vi "HatchManipulatorControl.Vi"(0 "Extend":bool, 1 "Slide":bool, 2 "Grip":bool, 3 "Pneumatics":T18={"Shifter"={"DevStatus"={"status"=FALSE, "code"=0, "source"=""}, "Pneumatics Control Module"=0, "Forward Solenoid Channel"=enum."Invalid", "Reverse Solenoid Channel"=enum."Invalid"}, "Compressor"={"DevStatus"={"status"=FALSE, "code"=0, "source"=""}, "Pneumatics Control Module"=0}, "Hatch Grip"={"DevStatus"={"status"=FALSE, "code"=0, "source"=""}, "Pneumatics Control Module"=0, "Forward Solenoid Channel"=enum."Invalid", "Reverse Solenoid Channel"=enum."Invalid"}, "Hatch Extend"={"DevStatus"={"status"=FALSE, "code"=0, "source"=""}, "Pneumatics Control Module"=0, "Forward Solenoid Channel"=enum."Invalid", "Reverse Solenoid Channel"=enum."Invalid"}, "Manipulator Slide"={"DevStatus"={"status"=FALSE, "code"=0, "source"=""}, "Pneumatics Control Module"=0, "Forward Solenoid Channel"=enum."Invalid", "Reverse Solenoid Channel"=enum."Invalid"}, "Hatch Floor Intake"={"DevStatus"={"status"=FALSE, "code"=0, "source"=""}, "Pneumatics Control Module"=0, "Forward Solenoid Channel"=enum."Invalid", "Reverse Solenoid Channel"=enum."Invalid"}}, 4 "RobotConfig":T1={"Motors"={"DriveRightPrimary"={"CAN Address"=1, "Invert"=FALSE, "InvertSensor"=FALSE, "Unit Conversion Factor"=0.0, "Brake Mode"=enum."Override to Brake", "Reverse Limt Switch Mode"=enum."Normally Closed", "Forward Limt Swith Mode"=enum."Normally Closed", "PWM Channel"=enum."Invalid", "Motor Controller Type"=enum."Talon SRX", "Peak Current (A)"=0, "Continuous Current (A)"=0, "Peak Duration (ms)"=0, "Current Limit Enable"=FALSE}, "DriveRightSecondary"={"CAN Address"=2, "Invert"=FALSE, "InvertSensor"=FALSE, "Unit Conversion Factor"=0.0, "Brake Mode"=enum."Override to Brake", "Reverse Limt Switch Mode"=enum."Normally Closed", "Forward Limt Swith Mode"=enum."Normally Closed", "PWM Channel"=enum."Invalid", "Motor Controller Type"=enum."Talon SRX", "Peak Current (A)"=0, "Continuous Current (A)"=0, "Peak Duration (ms)"=0, "Current Limit Enable"=FALSE}, "DriveLeftPrimary"={"CAN Address"=3, "Invert"=FALSE, "InvertSensor"=FALSE, "Unit Conversion Factor"=0.0, "Brake Mode"=enum."Override to Brake", "Reverse Limt Switch Mode"=enum."Normally Closed", "Forward Limt Swith Mode"=enum."Normally Closed", "PWM Channel"=enum."Invalid", "Motor Controller Type"=enum."Talon SRX", "Peak Current (A)"=0, "Continuous Current (A)"=0, "Peak Duration (ms)"=0, "Current Limit Enable"=FALSE}, "DriveLeftSecondary"={"CAN Address"=4, "Invert"=FALSE, "InvertSensor"=FALSE, "Unit Conversion Factor"=0.0, "Brake Mode"=enum."Override to Brake", "Reverse Limt Switch Mode"=enum."Normally Closed", "Forward Limt Swith Mode"=enum."Normally Closed", "PWM Channel"=enum."Invalid", "Motor Controller Type"=enum."Talon SRX", "Peak Current (A)"=0, "Continuous Current (A)"=0, "Peak Duration (ms)"=0, "Current Limit Enable"=FALSE}, "RearClimb"={"CAN Address"=8, "Invert"=FALSE, "InvertSensor"=FALSE, "Unit Conversion Factor"=0.0, "Brake Mode"=enum."Override to Brake", "Reverse Limt Switch Mode"=enum."Normally Closed", "Forward Limt Swith Mode"=enum."Normally Closed", "PWM Channel"=enum."Invalid", "Motor Controller Type"=enum."Talon SRX", "Peak Current (A)"=0, "Continuous Current (A)"=0, "Peak Duration (ms)"=0, "Current Limit Enable"=FALSE}, "Front Climb"={"CAN Address"=7, "Invert"=FALSE, "InvertSensor"=FALSE, "Unit Conversion Factor"=0.0, "Brake Mode"=enum."Override to Brake", "Reverse Limt Switch Mode"=enum."Normally Closed", "Forward Limt Swith Mode"=enum."Normally Closed", "PWM Channel"=enum."Invalid", "Motor Controller Type"=enum."Talon SRX", "Peak Current (A)"=0, "Continuous Current (A)"=0, "Peak Duration (ms)"=0, "Current Limit Enable"=FALSE}, "Climb Drive"={"CAN Address"=5, "Invert"=FALSE, "InvertSensor"=FALSE, "Unit Conversion Factor"=0.0, "Brake Mode"=enum."Override to Brake", "Reverse Limt Switch Mode"=enum."Normally Closed", "Forward Limt Swith Mode"=enum."Normally Closed", "PWM Channel"=enum."Invalid", "Motor Controller Type"=enum."Talon SRX", "Peak Current (A)"=0, "Continuous Current (A)"=0, "Peak Duration (ms)"=0, "Current Limit Enable"=FALSE}, "Shoulder1"={"CAN Address"=6, "Invert"=FALSE, "InvertSensor"=FALSE, "Unit Conversion Factor"=0.0, "Brake Mode"=enum."Override to Brake", "Reverse Limt Switch Mode"=enum."Normally Closed", "Forward Limt Swith Mode"=enum."Normally Closed", "PWM Channel"=enum."Invalid", "Motor Controller Type"=enum."Talon SRX", "Peak Current (A)"=0, "Continuous Current (A)"=0, "Peak Duration (ms)"=0, "Current Limit Enable"=FALSE}, "Shoulder2"={"CAN Address"=9, "Invert"=FALSE, "InvertSensor"=FALSE, "Unit Conversion Factor"=0.0, "Brake Mode"=enum."Override to Brake", "Reverse Limt Switch Mode"=enum."Normally Closed", "Forward Limt Swith Mode"=enum."Normally Closed", "PWM Channel"=enum."Invalid", "Motor Controller Type"=enum."Talon SRX", "Peak Current (A)"=0, "Continuous Current (A)"=0, "Peak Duration (ms)"=0, "Current Limit Enable"=FALSE}, "Wrist"={"CAN Address"=10, "Invert"=FALSE, "InvertSensor"=FALSE, "Unit Conversion Factor"=0.0, "Brake Mode"=enum."Override to Brake", "Reverse Limt Switch Mode"=enum."Disabled", "Forward Limt Swith Mode"=enum."Disabled", "PWM Channel"=enum."Invalid", "Motor Controller Type"=enum."Talon SRX", "Peak Current (A)"=0, "Continuous Current (A)"=0, "Peak Duration (ms)"=0, "Current Limit Enable"=FALSE}, "Extension"={"CAN Address"=11, "Invert"=FALSE, "InvertSensor"=FALSE, "Unit Conversion Factor"=0.0, "Brake Mode"=enum."Override to Brake", "Reverse Limt Switch Mode"=enum."Disabled", "Forward Limt Swith Mode"=enum."Disabled", "PWM Channel"=enum."Invalid", "Motor Controller Type"=enum."Talon SRX", "Peak Current (A)"=0, "Continuous Current (A)"=0, "Peak Duration (ms)"=0, "Current Limit Enable"=FALSE}, "CargoIntake"={"CAN Address"=11, "Invert"=FALSE, "InvertSensor"=FALSE, "Unit Conversion Factor"=0.0, "Brake Mode"=enum."Override to Brake", "Reverse Limt Switch Mode"=enum."Disabled", "Forward Limt Swith Mode"=enum."Disabled", "PWM Channel"=enum."Invalid", "Motor Controller Type"=enum."Talon SRX", "Peak Current (A)"=0, "Continuous Current (A)"=0, "Peak Duration (ms)"=0, "Current Limit Enable"=FALSE}, "Intake2"={"CAN Address"=11, "Invert"=FALSE, "InvertSensor"=FALSE, "Unit Conversion Factor"=0.0, "Brake Mode"=enum."Override to Brake", "Reverse Limt Switch Mode"=enum."Disabled", "Forward Limt Swith Mode"=enum."Disabled", "PWM Channel"=enum."Invalid", "Motor Controller Type"=enum."Talon SRX", "Peak Current (A)"=0, "Continuous Current (A)"=0, "Peak Duration (ms)"=0, "Current Limit Enable"=FALSE}}, "Sensors"={"IMU"={"Yaw Axis"=enum."Z", "SPI Bus"=enum."SPI MXP", "AHRS Algorithm"=enum."Complementary", "Calibration Time (s)"=3.0, "Calibrate On Open"=TRUE}, "HomingButton"={"DIOChannel"=enum."DIO 0", "Active Low"=FALSE}, "HomingLED_Green"={"DIOChannel"=enum."DIO 0", "Active Low"=FALSE}, "HomingLED_Yellow"={"DIOChannel"=enum."DIO 0", "Active Low"=FALSE}, "HomingLED_Red"={"DIOChannel"=enum."DIO 0", "Active Low"=FALSE}}, "PID"={"FrontClimb"={"P"=0.0, "I"=0.0, "D"=0.0, "F"=0.0, "IZone"=0.0}, "RearClimb"={"P"=0.0, "I"=0.0, "D"=0.0, "F"=0.0, "IZone"=0.0}, "ArmShoulder"={"P"=0.0, "I"=0.0, "D"=0.0, "F"=0.0, "IZone"=0.0}, "ArmExtend"={"P"=0.0, "I"=0.0, "D"=0.0, "F"=0.0, "IZone"=0.0}, "ArmWrist"={"P"=0.0, "I"=0.0, "D"=0.0, "F"=0.0, "IZone"=0.0}}, "Solenoids"={" Shifter"={"SolenoidChannel"=enum."Solenoid 3", "Invert"=FALSE}, "Hatch Grip"={"SolenoidChannel"=enum."Solenoid 0", "Invert"=FALSE}, "Hatch Extend"={"SolenoidChannel"=enum."Solenoid 0", "Invert"=FALSE}, "Manipulator Slide"={"SolenoidChannel"=enum."Solenoid 0", "Invert"=FALSE}, "Hatch Floor Intake"={"SolenoidChannel"=enum."Solenoid 0", "Invert"=FALSE}}, "Enable Compressor"=TRUE, "MotionMagic"={"FrontClimbExtend"={"CruiseVelocity"=0, "Acceleration"=0}, "RearClimbExtend"={"CruiseVelocity"=0, "Acceleration"=0}, "FrontClimbRetract"={"CruiseVelocity"=0, "Acceleration"=0}, "RearClimbRetract"={"CruiseVelocity"=0, "Acceleration"=0}}, "RobotDimensions"={"Length (in)"=0.0, "Shoulder Height (in)"=0.0, "Frame Height (in)"=0.0, "Arm Center to Front of Robot (in)"=0.0, "Arm Min Extension (in)"=0.0, "Arm Max Extension (in)"=0.0, "Cargo Intake Loop Length (in)"=0.0, "Cargo Intake Loop Width (in)"=0.0, "Cargo Intake Loop Offset (in)"=0.0, "Cargo Intake Loop Angle (rad)"=0.0}, "Arm Home Position"={"Radius (in)"=0.0, "ShoulderAngle (rad)"=0.0, "WristAngle (rad)"=0.0}, "Climb Home Position"={"Back Climb"=0.0, "Front Climb"=0.0}, "Climb Positions"={"Retract"=0.0, "Level 2"=0.0, "Level 3"=0.0}}) -> ()   [LabVIEW 2019]
uses:
  TypeDefs/RobotComponents/RobotPneumatics.ctl
  <vilib>/Rock Robotics/WPI/Solenoid/WPI_SolenoidDevRef.ctl
  <vilib>/Rock Robotics/WPI/Solenoid/WPI_SolenoidChannel.ctl
  <vilib>/Rock Robotics/WPI/Compressor/WPI_CompressorDevRef.ctl
  TypeDefs/ConfigComponents/Config_Robot.ctl
  ArgosLib/Config/ConfigComponents/TypeDefs/Config_Motor.ctl
  <vilib>/Rock Robotics/WPI/ThirdParty/Phoenix-LabVIEW/Motor Controller/Controls/CTRE_Phoenix_MotorControl_NeutralMode.ctl
  <vilib>/Rock Robotics/WPI/ThirdParty/Phoenix-LabVIEW/Motor Controller/Controls/CTRE_Phoenix_MotorControl_LimitSwitchNormal.ctl
  <vilib>/Rock Robotics/SystemInterfaces/DIO/FPGA_DIOPWMChannel.ctl
  ArgosLib/Config/ConfigComponents/TypeDefs/Config_MotorCtrlType.ctl
  ArgosLib/Config/ConfigComponents/TypeDefs/Config_IMU.ctl
  <vilib>/Rock Robotics/SystemInterfaces/spilib/spi_bus.ctl
  ArgosLib/Config/ConfigComponents/TypeDefs/Config_DigitalIO.ctl
  <vilib>/Rock Robotics/SystemInterfaces/DIO/FPGA_DIOChannel.ctl
  ArgosLib/Config/ConfigComponents/TypeDefs/Config_PIDParams.ctl
  ArgosLib/Config/ConfigComponents/TypeDefs/Config_SingleSolenoid.ctl
  ArgosLib/Config/ConfigComponents/TypeDefs/Config_MotionMagicParams.ctl
  TypeDefs/ConfigComponents/Config_Dimensions.ctl
  Arm/TypeDefs/ArmCoordinate.ctl
  Climber/TypeDefs/ClimberPositionHeights.ctl
  <vilib>/Rock Robotics/WPI/Solenoid/WPI_SolenoidValue.ctl
  <vilib>/Rock Robotics/WPI/Solenoid/WPI_SolenoidSetEnum.vi
  ArgosLib/ArgosLib.lvlib
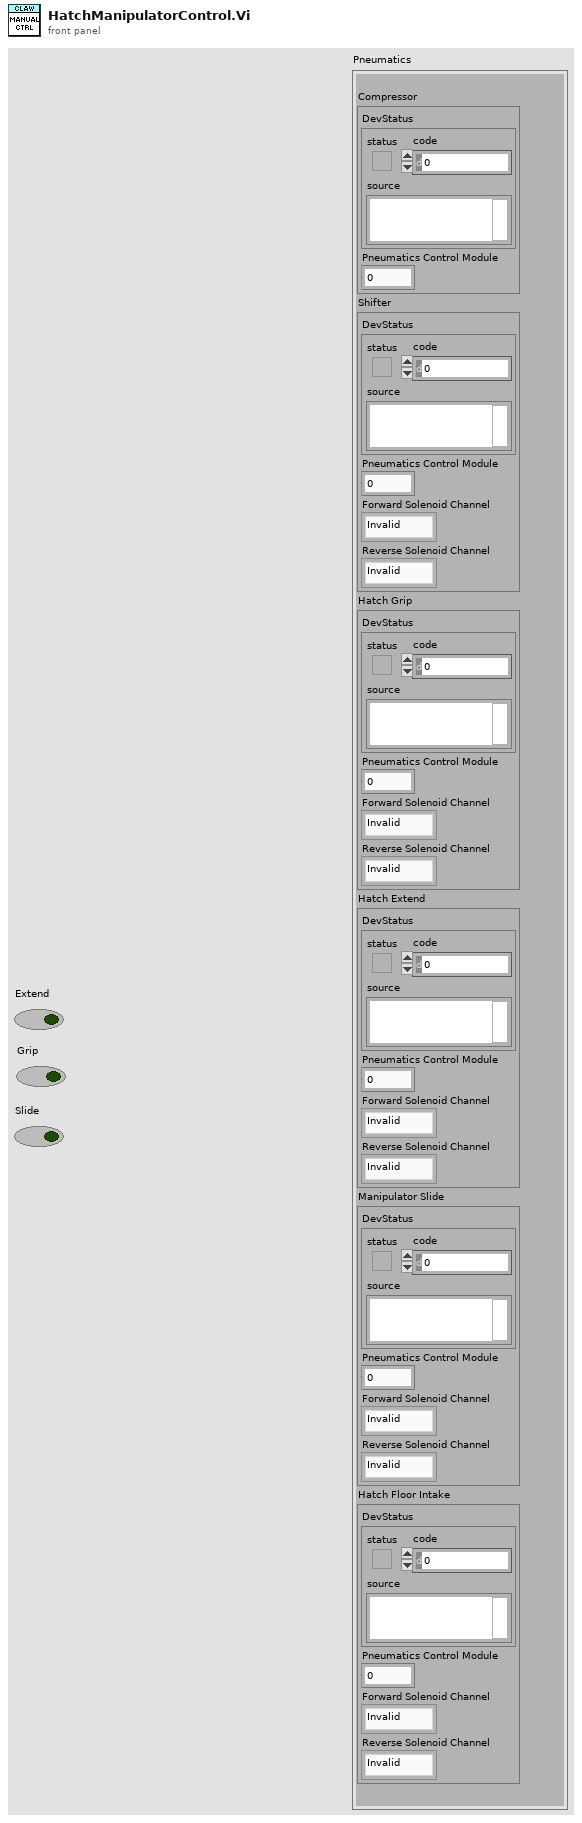
[diagram p1: front panel]
types:
  T1 = typedef "Config_Robot.ctl" = cluster{"Motors":cluster{"DriveRightPrimary":T2, "DriveRightSecondary":T2, "DriveLeftPrimary":T2, "DriveLeftSecondary":T2, "RearClimb":T2, "Front Climb":T2, "Climb Drive":T2, "Shoulder1":T2, "Shoulder2":T2, "Wrist":T2, "Extension":T2, "CargoIntake":T2, "Intake2":T2}, "Sensors":cluster{"IMU":T7, "HomingButton":T9, "HomingLED_Green":T9, "HomingLED_Yellow":T9, "HomingLED_Red":T9}, "PID":cluster{"FrontClimb":T11, "RearClimb":T11, "ArmShoulder":T11, "ArmExtend":T11, "ArmWrist":T11}, "Solenoids":cluster{" Shifter":T12, "Hatch Grip":T12, "Hatch Extend":T12, "Manipulator Slide":T12, "Hatch Floor Intake":T12}, "Enable Compressor":bool, "MotionMagic":cluster{"FrontClimbExtend":T14, "RearClimbExtend":T14, "FrontClimbRetract":T14, "RearClimbRetract":T14}, "RobotDimensions":T15, "Arm Home Position":T16, "Climb Home Position":cluster{"Back Climb":dbl, "Front Climb":dbl}, "Climb Positions":T17}
  T2 = typedef "ArgosLib.lvlib/Config_Motor.ctl" = cluster{"CAN Address":u8, "Invert":bool, "InvertSensor":bool, "Unit Conversion Factor":dbl, "Brake Mode":T3, "Reverse Limt Switch Mode":T4, "Forward Limt Swith Mode":T4, "PWM Channel":T5, "Motor Controller Type":T6, "Peak Current (A)":i32, "Continuous Current (A)":i32, "Peak Duration (ms)":i32, "Current Limit Enable":bool}
  T3 = typedef "CTRE_Phoenix_MotorControl_NeutralMode.ctl" = enum8{"EEPROMSetting", "Override to Coast", "Override to Brake"}
  T4 = typedef "CTRE_Phoenix_MotorControl_LimitSwitchNormal.ctl" = enum16{"Normally Open", "Normally Closed", "Disabled"}
  T5 = typedef "FPGA_DIOPWMChannel.ctl" = enum8{"PWM 0", "PWM 1", "PWM 2", "PWM 3", "PWM 4", "PWM 5", "PWM 6", "PWM 7", "PWM 8", "PWM 9", "PWM MXP 0", "PWM MXP 1", "PWM MXP 2", "PWM MXP 3", "PWM MXP 4", "PWM MXP 5", "PWM MXP 6", "PWM MXP 7", "PWM MXP 8", "PWM MXP 9", "Invalid"}
  T6 = typedef "ArgosLib.lvlib/Config_MotorCtrlType.ctl" = enum16{"Disabled", "Talon SRX", "Talon SR", "Venom"}
  T7 = typedef "ArgosLib.lvlib/Config_IMU.ctl" = cluster{"Yaw Axis":enum16{"X", "Y", "Z"}, "SPI Bus":T8, "AHRS Algorithm":enum16{"Complementary", "Madgwick"}, "Calibration Time (s)":dbl, "Calibrate On Open":bool}
  T8 = typedef "spi_bus.ctl" = enum16{"SPI On-Board, CS0", "SPI On-Board, CS1", "SPI On-Board, CS2", "SPI On-Board, CS3", "SPI MXP", "Invalid"}
  T9 = typedef "ArgosLib.lvlib/Config_DigitalIO.ctl" = cluster{"DIOChannel":T10, "Active Low":bool}
  T10 = typedef "FPGA_DIOChannel.ctl" = enum8{"DIO 0", "DIO 1", "DIO 2", "DIO 3", "DIO 4", "DIO 5", "DIO 6", "DIO 7", "DIO 8", "DIO 9", "DIO MXP 0", "DIO MXP 1", "DIO MXP 2", "DIO MXP 3", "DIO MXP 4", "DIO MXP 5", "DIO MXP 6", "DIO MXP 7", "DIO MXP 8", "DIO MXP 9", "DIO MXP 10", "DIO MXP 11", "DIO MXP 12", "DIO MXP 13", "DIO MXP 14", "DIO MXP 15", "SPI Port CS1", "SPI Port CS2", "SPI Port CS3", "SPI Port MISO", "SPI Port MOSI", "Invalid"}
  T11 = typedef "ArgosLib.lvlib/Config_PIDParams.ctl" = cluster{"P":dbl, "I":dbl, "D":dbl, "F":dbl, "IZone":dbl}
  T12 = typedef "ArgosLib.lvlib/Config_SingleSolenoid.ctl" = cluster{"SolenoidChannel":T13, "Invert":bool}
  T13 = typedef "WPI_SolenoidChannel.ctl" = enum8{"Solenoid 0", "Solenoid 1", "Solenoid 2", "Solenoid 3", "Solenoid 4", "Solenoid 5", "Solenoid 6", "Solenoid 7", "Invalid"}
  T14 = typedef "Config_MotionMagicParams.ctl" = cluster{"CruiseVelocity":i32, "Acceleration":i32}
  T15 = typedef "Config_Dimensions.ctl" = cluster{"Length (in)":dbl, "Shoulder Height (in)":dbl, "Frame Height (in)":dbl, "Arm Center to Front of Robot (in)":dbl, "Arm Min Extension (in)":dbl, "Arm Max Extension (in)":dbl, "Cargo Intake Loop Length (in)":dbl, "Cargo Intake Loop Width (in)":dbl, "Cargo Intake Loop Offset (in)":dbl, "Cargo Intake Loop Angle (rad)":dbl}
  T16 = typedef "ArmCoordinate.ctl" = cluster{"Radius (in)":dbl, "ShoulderAngle (rad)":dbl, "WristAngle (rad)":dbl}
  T17 = typedef "ClimberPositionHeights.ctl" = cluster{"Retract":dbl, "Level 2":dbl, "Level 3":dbl}
  T18 = typedef "RobotPneumatics.ctl" = cluster{"Shifter":T19, "Compressor":T20, "Hatch Grip":T19, "Hatch Extend":T19, "Manipulator Slide":T19, "Hatch Floor Intake":T19}
  T19 = typedef "WPI_SolenoidDevRef.ctl" = cluster{"DevStatus":errorcluster, "Pneumatics Control Module":u8, "Forward Solenoid Channel":T13, "Reverse Solenoid Channel":T13}
  T20 = typedef "WPI_CompressorDevRef.ctl" = cluster{"DevStatus":errorcluster, "Pneumatics Control Module":u8}
  T21 = typedef "WPI_SolenoidValue.ctl" = enum16{"Off", "On", "Forward", "Reverse"}
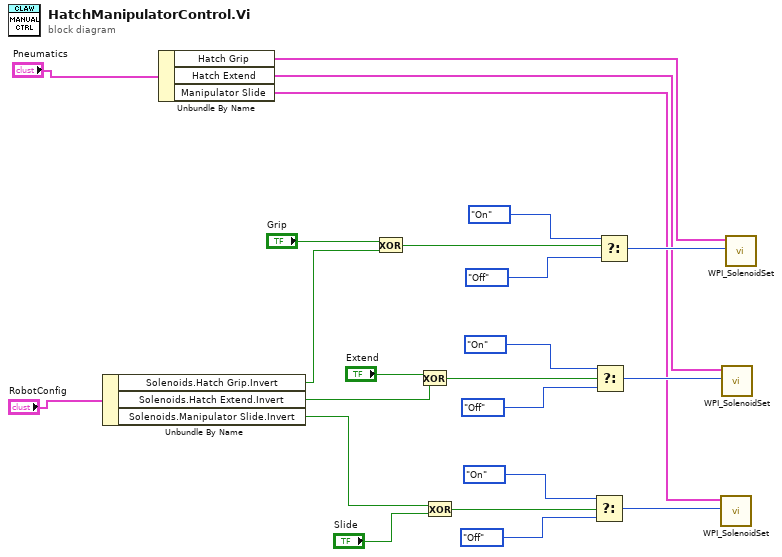
[diagram p0: block diagram]
diagram:
  n1 = Unbundle By Name("RobotConfig") -> ("Solenoids.Hatch Grip.Invert"=w10:bool, "Solenoids.Hatch Extend.Invert"=w7:bool, "Solenoids.Manipulator Slide.Invert"=w20:bool)
  n2 = Unbundle By Name("Pneumatics") -> ("Hatch Grip"=w3:T19, "Hatch Extend"=w2:T19, "Manipulator Slide"=w1:T19)
  n3 = Exclusive Or(1:w10, 2:"Grip") -> (0:w8:bool)
  n4 = Exclusive Or(1:w7, 2:"Extend") -> (0:w5:bool)
  n5 = Exclusive Or(1:"Slide", 2:w20) -> (0:w4:bool)
  n6 = Select(t=WPI_SolenoidValue."On" ("Value"), s=w4, f=WPI_SolenoidValue."Off") -> (s? t:f=w12:T21)
  n7 = Select(t=WPI_SolenoidValue."On" ("Value"), s=w5, f=WPI_SolenoidValue."Off") -> (s? t:f=w15:T21)
  n8 = Select(t=WPI_SolenoidValue."On" ("Value"), s=w8, f=WPI_SolenoidValue."Off") -> (s? t:f=w17:T21)
  n9 = call-poly <vilib>:"WPI_SolenoidSet.vi"("Value"=w12, "SolenoidDevRef"=w1) -> ()  [unwired: 8 in, 2 out]
  n10 = call-poly <vilib>:"WPI_SolenoidSet.vi"("Value"=w15, "SolenoidDevRef"=w2) -> ()  [unwired: 8 in, 2 out]
  n11 = call-poly <vilib>:"WPI_SolenoidSet.vi"("Value"=w17, "SolenoidDevRef"=w3) -> ()  [unwired: 8 in, 2 out]
